vi "Accessors Loopback Test.vi"() -> ()   [LabVIEW 2021]
uses:
  Class/CIFCorePlugin.lvclass
  Class/CIFCorePlugin.lvclass/CIFCorePlugin.ctl
  Class/Typedef/Running Internal Data.ctl
  Common/Typedef/Timing Overrides.ctl
  Common/Typedef/Common Plugin Configuration.ctl
  Common/Typedef/External Clock Config.ctl
  Class/Accessors/Monitor/Write Double 1.vi
  Class/Accessors/Monitor/Write Double 2.vi
  Class/Accessors/Monitor/Write Double 3.vi
  Class/Accessors/Monitor/Write Double 4.vi
  Class/Accessors/Monitor/Write I64 1.vi
  Class/Accessors/Monitor/Write I64 2.vi
  Class/Accessors/Monitor/Write I64 3.vi
  Class/Accessors/Monitor/Write I64 4.vi
  Class/Accessors/Monitor/Write U64 1.vi
  Class/Accessors/Monitor/Write U64 2.vi
  Class/Accessors/Monitor/Write U64 3.vi
  Class/Accessors/Monitor/Write U64 4.vi
  Class/Accessors/Monitor/Read Double 1.vi
  Class/Accessors/Monitor/Read Double 2.vi
  Class/Accessors/Monitor/Read Double 3.vi
  Class/Accessors/Monitor/Read Double 4.vi
  Class/Accessors/Monitor/Read I64 1.vi
  Class/Accessors/Monitor/Read I64 2.vi
  Class/Accessors/Monitor/Read I64 3.vi
  Class/Accessors/Monitor/Read I64 4.vi
  Class/Accessors/Monitor/Read U64 1.vi
  Class/Accessors/Monitor/Read U64 2.vi
  Class/Accessors/Monitor/Read U64 3.vi
  Class/Accessors/Monitor/Read U64 4.vi
  Class/Accessors/Timestamps/Write Cleanup TS.vi
  Class/Accessors/Timestamps/Write Creation TS.vi
  Class/Accessors/Timestamps/Write Destoying TS.vi
  Class/Accessors/Timestamps/Write Housekeeping TS.vi
  Class/Accessors/Timestamps/Write Listening TS.vi
  Class/Accessors/Timestamps/Write R-FIFO TS.vi
  Class/Accessors/Timestamps/Write Sleep TS.vi
  Class/Accessors/Timestamps/Write Target Wake TS.vi
  Class/Accessors/Timestamps/Write W-Output TS.vi
  Class/Accessors/Timestamps/Write Execute TS.vi
  Class/Accessors/Timestamps/Read Cleanup TS.vi
  Class/Accessors/Timestamps/Read Creation TS.vi
  Class/Accessors/Timestamps/Read Destroying TS.vi
  Class/Accessors/Timestamps/Read Housekeeping TS.vi
  Class/Accessors/Timestamps/Read Listening TS.vi
  Class/Accessors/Timestamps/Read R-FIFO TS.vi
  Class/Accessors/Timestamps/Read Sleep TS.vi
  Class/Accessors/Timestamps/Read Target Wake TS.vi
  Class/Accessors/Timestamps/Read W-Output TS.vi
  Class/Accessors/Timestamps/Read Execute TS.vi
  Class/Accessors/Write Running Internal Data.vi
  Class/Accessors/Write Timing Override.vi
  Class/Accessors/Read Running Internal Data.vi
  Class/Accessors/Read Timing Override.vi
  Class/Accessors/Read Common Config.vi
  <vilib>/CIF Foundation/CIF Utilities/Time/System Time/Get System Time.vi
  Class/Logs/Log State Change.vi
  Common/CIFCoreCommon.lvlib
panel:
  out "status":string
  out "pass":bool
  out "error out":errorcluster
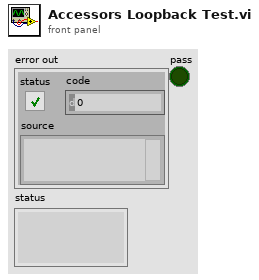
[diagram p1: front panel]
types:
  T1 = cluster{"Monitor dbl1":dbl, "Monitor dbl2":dbl, "Monitor dbl3":dbl, "Monitor dbl4":dbl, "Monitor i64 1":i64, "Monitor i64 2":i64, "Monitor i64 3":i64, "Monitor i64 4":i64, "Monitor u64 1":u64, "Monitor u64 2":u64, "Monitor u64 3":u64, "Monitor u64 4":u64}
  T2 = cluster{"TS Cleanup":u64, "TS Creation":u64, "TS Destroying":u64, "TS Housekeeping":u64, "TS Listening":u64, "TS Read FIFO":u64, "TS Sleep":u64, "TS Target Wake":u64, "TS Write Output":u64, "TSExecute":u64}
  T3 = typedef "CIFCorePlugin.lvclass/Running Internal Data.ctl" = cluster{"Refresh":bool, "Iterations":i64, "Housekeep only":bool, "Configured period (ns)":i64, "Update channel OOB":bool, "Configuration Change":bool, "Disable Auto Benchmark":bool, "gRPC Loop":bool, "Timed Loop Supported":bool, "Windows Late Cycle Warning":bool}
  T4 = typedef "CIFCoreCommon.lvlib/Timing Overrides.ctl" = cluster{"Override Timing":bool, "Skip Sleep":bool, "Period (s)":dbl}
  T5 = typedef "CIFCoreCommon.lvlib/Common Plugin Configuration.ctl" = cluster{"Period (s)":dbl, "Offset (us)":i32, "Priority":i32, "Processor":i32, "External Clock":T6}
  T6 = typedef "CIFCoreCommon.lvlib/External Clock Config.ctl" = cluster{"ClockID":u8, "Clock Name":string, "Publish Clock":bool, "Convert Data Timestamps":bool, "Plugin Timing Source":bool}
  T7 = cluster{"Running Internal Data":T3, "Timing Override":T4, "Common Configuration":T5}
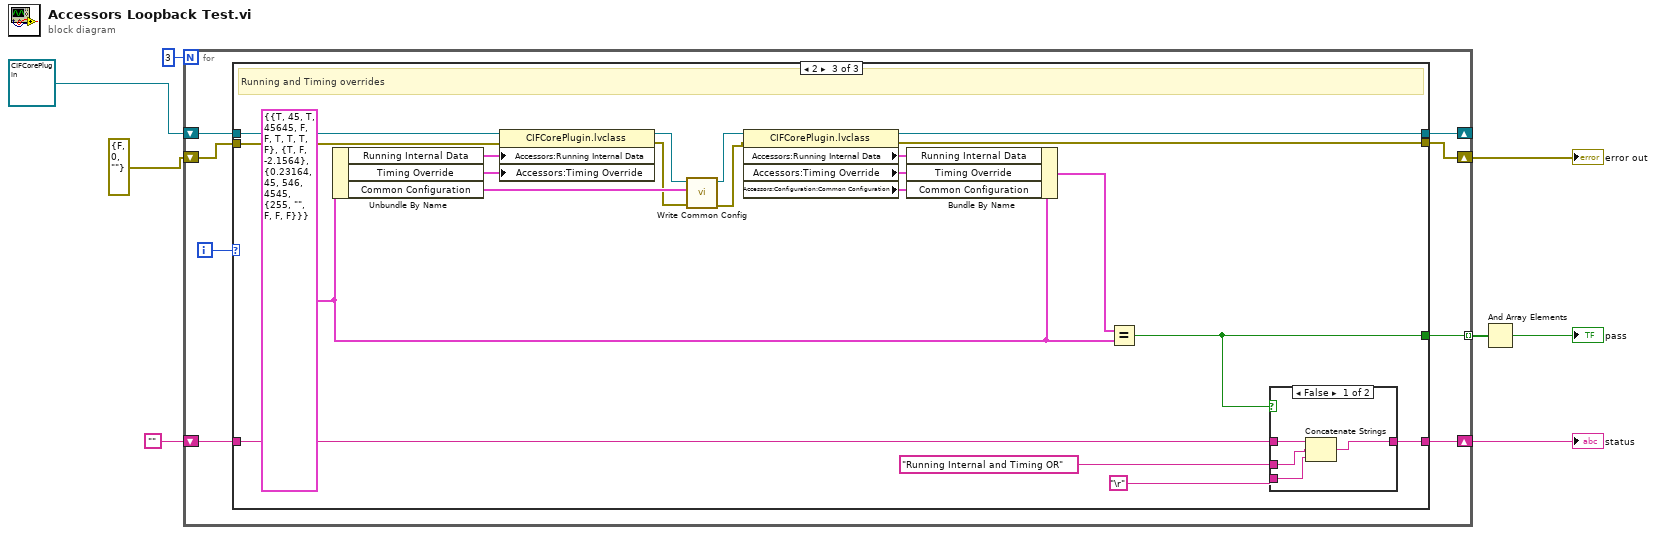
[diagram p0: block diagram]
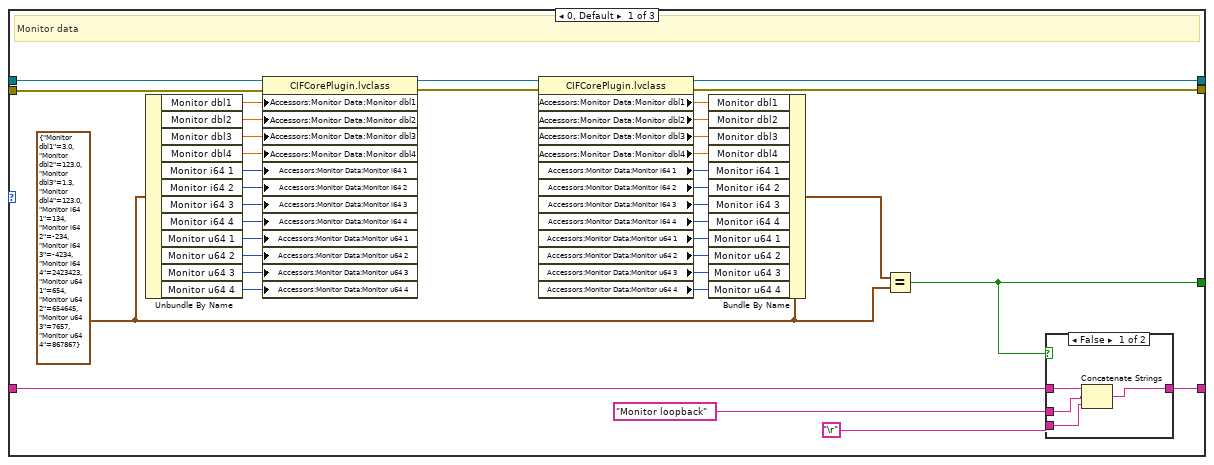
[diagram p2: hidden frame]
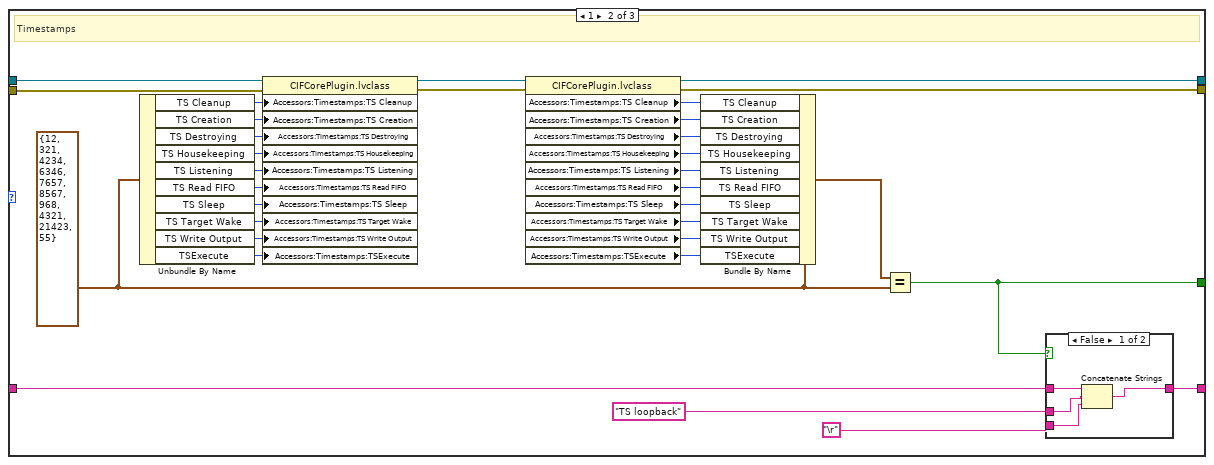
[diagram p4: hidden frame]
diagram:
  n1 = for {
    N: 3 -> [_]
    tunnel: [w16] -> w8 mode=indexing
    shift-right: [w13] -> w1
    shift-left: errorcluster {"status"=FALSE, "code"=0, "source"=""} ("error out") -> [w15]
    shift-right: [w11] -> _
    shift-left: refnum<class "CIFCorePlugin.lvclass"> refnum ("CIFCorePlugin.lvclass") -> [w14]
    shift-right: [w9] -> w5
    shift-left: "" -> [w10]
    i -> [w12]
    n2 = case shown="2" w12 {
      tunnel: [w17 w81 w108] -> w16
      tunnel: w15 -> [w48 w86 w112]
      tunnel: w14 -> [w49 w87 w113]
      tunnel: [w44 w82 w110] -> w13
      tunnel: [w45 w83 w111] -> w11
      tunnel: w10 -> [w53 w91 w117]
      tunnel: [w52 w90 w116] -> w9
      frame 0, Default {
        w18 = T1 {"Monitor dbl1"=3.0, "Monitor dbl2"=123.0, "Monitor dbl3"=1.3, "Monitor dbl4"=123.0, "Monitor i64 1"=134, "Monitor i64 2"=-234, "Monitor i64 3"=-4234, "Monitor i64 4"=2423423, "Monitor u64 1"=654, "Monitor u64 2"=654645, "Monitor u64 3"=7657, "Monitor u64 4"=867867}
        # "Monitor data"
        n3 = Unbundle By Name(w18) -> ("Monitor dbl1"=w32:dbl, "Monitor dbl2"=w33:dbl, "Monitor dbl3"=w34:dbl, "Monitor dbl4"=w35:dbl, "Monitor i64 1"=w36:i64, "Monitor i64 2"=w37:i64, "Monitor i64 3"=w38:i64, "Monitor i64 4"=w39:i64, "Monitor u64 1"=w40:u64, "Monitor u64 2"=w41:u64, "Monitor u64 3"=w42:u64, "Monitor u64 4"=w43:u64)
        n4 = property class="CIFCorePlugin.lvclass"(reference=w49, error in=w48, "Accessors:Monitor Data:Monitor dbl1"=w32, "Accessors:Monitor Data:Monitor dbl2"=w33, "Accessors:Monitor Data:Monitor dbl3"=w34, "Accessors:Monitor Data:Monitor dbl4"=w35, "Accessors:Monitor Data:Monitor i64 1"=w36, "Accessors:Monitor Data:Monitor i64 2"=w37, "Accessors:Monitor Data:Monitor i64 3"=w38, "Accessors:Monitor Data:Monitor i64 4"=w39, "Accessors:Monitor Data:Monitor u64 1"=w40, "Accessors:Monitor Data:Monitor u64 2"=w41, "Accessors:Monitor Data:Monitor u64 3"=w42, "Accessors:Monitor Data:Monitor u64 4"=w43) -> (reference out=w47:refnum<class "CIFCorePlugin.lvclass">, error out=w46:errorcluster)
        n5 = property class="CIFCorePlugin.lvclass"(reference=w47, error in=w46) -> (reference out=w45:refnum<class "CIFCorePlugin.lvclass">, error out=w44:errorcluster, "Accessors:Monitor Data:Monitor dbl1"=w31:dbl, "Accessors:Monitor Data:Monitor dbl2"=w20:dbl, "Accessors:Monitor Data:Monitor dbl3"=w21:dbl, "Accessors:Monitor Data:Monitor dbl4"=w22:dbl, "Accessors:Monitor Data:Monitor i64 1"=w23:i64, "Accessors:Monitor Data:Monitor i64 2"=w24:i64, "Accessors:Monitor Data:Monitor i64 3"=w25:i64, "Accessors:Monitor Data:Monitor i64 4"=w26:i64, "Accessors:Monitor Data:Monitor u64 1"=w27:u64, "Accessors:Monitor Data:Monitor u64 2"=w28:u64, "Accessors:Monitor Data:Monitor u64 3"=w29:u64, "Accessors:Monitor Data:Monitor u64 4"=w30:u64)
        n6 = Bundle By Name(cluster=w18, "Monitor dbl1"=w31, "Monitor dbl2"=w20, "Monitor dbl3"=w21, "Monitor dbl4"=w22, "Monitor i64 1"=w23, "Monitor i64 2"=w24, "Monitor i64 3"=w25, "Monitor i64 4"=w26, "Monitor u64 1"=w27, "Monitor u64 2"=w28, "Monitor u64 3"=w29, "Monitor u64 4"=w30) -> (w19:T1)
        n7 = Equal?(x=w19, y=w18) -> (x = y?=w17:bool)
        n8 = case shown="False" w17 {
          tunnel: w53 -> [w57 w58]
          tunnel: [w54 w58] -> w52
          tunnel: "Monitor loopback" -> [w56 _]
          tunnel: "\r" -> [w55 _]
          frame False {
            n9 = Concatenate Strings(w57, w56, w55) -> (w54:string)
          }
          frame True {
          }
        }
      }
      frame 1 {
        w59 = T2 {"TS Cleanup"=12, "TS Creation"=321, "TS Destroying"=4234, "TS Housekeeping"=6346, "TS Listening"=7657, "TS Read FIFO"=8567, "TS Sleep"=968, "TS Target Wake"=4321, "TS Write Output"=21423, "TSExecute"=55}
        # "Timestamps"
        n10 = Unbundle By Name(w59) -> ("TS Cleanup"=w80:u64, "TS Creation"=w71:u64, "TS Destroying"=w72:u64, "TS Housekeeping"=w73:u64, "TS Listening"=w74:u64, "TS Read FIFO"=w75:u64, "TS Sleep"=w76:u64, "TS Target Wake"=w77:u64, "TS Write Output"=w78:u64, "TSExecute"=w79:u64)
        n11 = property class="CIFCorePlugin.lvclass"(reference=w87, error in=w86, "Accessors:Timestamps:TS Cleanup"=w80, "Accessors:Timestamps:TS Creation"=w71, "Accessors:Timestamps:TS Destroying"=w72, "Accessors:Timestamps:TS Housekeeping"=w73, "Accessors:Timestamps:TS Listening"=w74, "Accessors:Timestamps:TS Read FIFO"=w75, "Accessors:Timestamps:TS Sleep"=w76, "Accessors:Timestamps:TS Target Wake"=w77, "Accessors:Timestamps:TS Write Output"=w78, "Accessors:Timestamps:TSExecute"=w79) -> (reference out=w85:refnum<class "CIFCorePlugin.lvclass">, error out=w84:errorcluster)
        n12 = property class="CIFCorePlugin.lvclass"(reference=w85, error in=w84) -> (reference out=w83:refnum<class "CIFCorePlugin.lvclass">, error out=w82:errorcluster, "Accessors:Timestamps:TS Cleanup"=w61:i64, "Accessors:Timestamps:TS Creation"=w62:i64, "Accessors:Timestamps:TS Destroying"=w63:i64, "Accessors:Timestamps:TS Housekeeping"=w64:i64, "Accessors:Timestamps:TS Listening"=w65:i64, "Accessors:Timestamps:TS Read FIFO"=w66:i64, "Accessors:Timestamps:TS Sleep"=w67:i64, "Accessors:Timestamps:TS Target Wake"=w68:i64, "Accessors:Timestamps:TS Write Output"=w69:i64, "Accessors:Timestamps:TSExecute"=w70:i64)
        n13 = Bundle By Name(cluster=w59, "TS Cleanup"=w61, "TS Creation"=w62, "TS Destroying"=w63, "TS Housekeeping"=w64, "TS Listening"=w65, "TS Read FIFO"=w66, "TS Sleep"=w67, "TS Target Wake"=w68, "TS Write Output"=w69, "TSExecute"=w70) -> (w60:T2)
        n14 = Equal?(x=w60, y=w59) -> (x = y?=w81:bool)
        n15 = case shown="False" w81 {
          tunnel: w91 -> [w95 w96]
          tunnel: [w92 w96] -> w90
          tunnel: "TS loopback" -> [w94 _]
          tunnel: "\r" -> [w93 _]
          frame False {
            n16 = Concatenate Strings(w95, w94, w93) -> (w92:string)
          }
          frame True {
          }
        }
      }
      frame 2 {
        w105 = T7 {"Running Internal Data"={"Refresh"=TRUE, "Iterations"=45, "Housekeep only"=TRUE, "Configured period (ns)"=45645, "Update channel OOB"=FALSE, "Configuration Change"=FALSE, "Disable Auto Benchmark"=TRUE, "gRPC Loop"=TRUE, "Timed Loop Supported"=TRUE, "Windows Late Cycle Warning"=FALSE}, "Timing Override"={"Override Timing"=TRUE, "Skip Sleep"=FALSE, "Period (s)"=-2.1564}, "Common Configuration"={"Period (s)"=0.23164, "Offset (us)"=45, "Priority"=546, "Processor"=4545, "External Clock"={"ClockID"=255, "Clock Name"="", "Publish Clock"=FALSE, "Convert Data Timestamps"=FALSE, "Plugin Timing Source"=FALSE}}}
        # "Running and Timing overrides"
        n17 = Unbundle By Name(w105) -> ("Running Internal Data"=w107:T3, "Timing Override"=w106:T4, "Common Configuration"=w99:T5)
        n18 = property class="CIFCorePlugin.lvclass"(reference=w113, error in=w112, "Accessors:Running Internal Data"=w107, "Accessors:Timing Override"=w106) -> (reference out=w101:refnum<class "CIFCorePlugin.lvclass">, error out=w98:errorcluster)
        n19 = call "Write Common Config.vi"("error in (no error)"=w98, "Common"=w99, "CIFTemplateNode in"=w101) -> ("error out"=w97:errorcluster, "CIFTemplateNode out"=w100:refnum<class "CIFCorePlugin.lvclass">)  [unwired: 7 in]
        n20 = property class="CIFCorePlugin.lvclass"(reference=w100, error in=w97) -> (reference out=w111:refnum<class "CIFCorePlugin.lvclass">, error out=w110:errorcluster, "Accessors:Running Internal Data"=w104:T3, "Accessors:Timing Override"=w103:T4, "Accessors:Configuration:Common Configuration"=w102:T5)
        n21 = Bundle By Name(cluster=w105, "Running Internal Data"=w104, "Timing Override"=w103, "Common Configuration"=w102) -> (w109:T7)
        n22 = Equal?(x=w109, y=w105) -> (x = y?=w108:bool)
        n23 = case shown="False" w108 {
          tunnel: w117 -> [w121 w122]
          tunnel: [w118 w122] -> w116
          tunnel: "Running Internal and Timing OR" -> [w120 _]
          tunnel: "\r" -> [w119 _]
          frame False {
            n24 = Concatenate Strings(w121, w120, w119) -> (w118:string)
          }
          frame True {
          }
        }
      }
    }
  }
  "error out" <- w1
  "status" <- w5
  n25 = And Array Elements(Boolean array=w8) -> (logical AND=→"pass":bool)
